vi "Day 5.vi"() -> ()   [LabVIEW 2019]
panel:
  out "Total Time":dbl
  out "Minimize Polymer Time":dbl
  out "React Polymer Time":dbl
  out "Read File Time":dbl
  out "Redux Polymer":string
  out "Error Out":errorcluster
  out "Length of Shortest Polymer":i32
  out "Element Creating Shortest Polymer":string
  out "Polymer Length":i32
  out "Polymer After Reacting":string
  in  "error in (no error)":errorcluster
  in  "Use Example Input":bool
  in  "Example Input":string="dabAcCaCBAcCcaDA"
  in  "Relative Path to Input File":string="Day 5\\Day 5 Raw Input.txt"
  # "Part 1"
  # "Part 2"
  # "~0.43 s is fastest time"
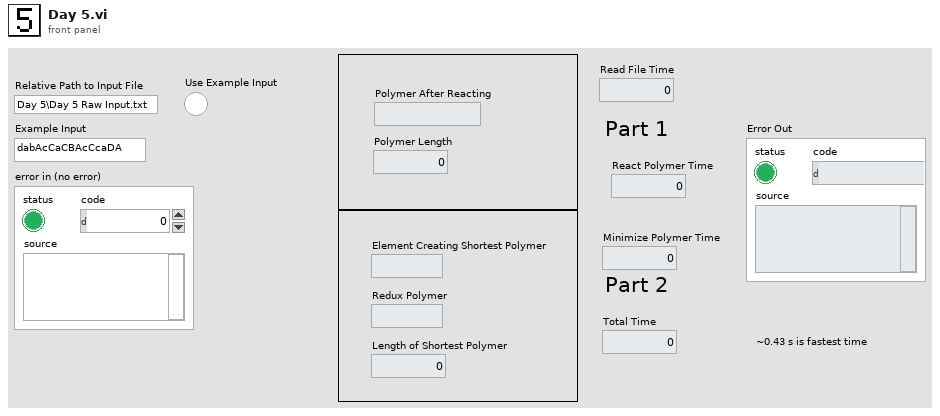
[diagram p1: front panel]
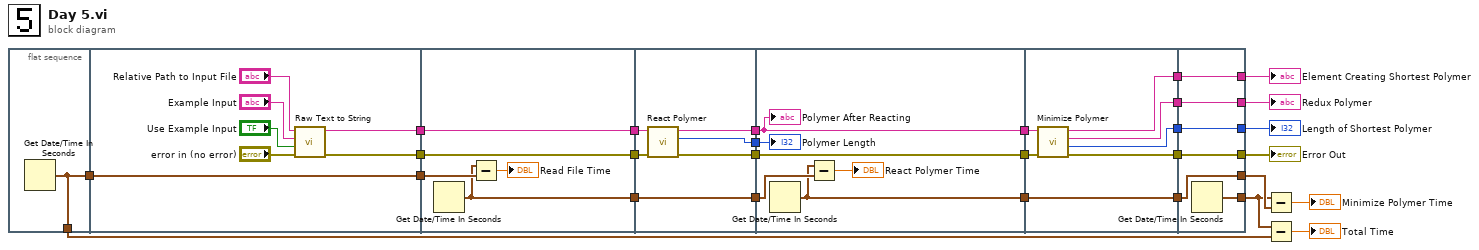
[diagram p0: block diagram]
diagram:
  n1 = flat-sequence {
    tunnel: [w29] -> w28
    tunnel: [w29] -> w9
    tunnel: w28 -> [w36]
    tunnel: [w36] -> w27
    tunnel: [w31] -> w20
    tunnel: [w30] -> w17
    tunnel: w27 -> [w40]
    tunnel: [w39] -> w26
    tunnel: [w38] -> w21
    tunnel: w20 -> [w38]
    tunnel: w17 -> [w37]
    tunnel: [w37] -> w16
    tunnel: w26 -> [w47]
    tunnel: [w47] -> w25
    tunnel: w21 -> [w46]
    tunnel: [w45] -> w19
    tunnel: w16 -> [w44]
    tunnel: [w43] -> w11
    tunnel: [w42] -> w10
    tunnel: w25 -> [w53]
    tunnel: [w51] -> w24
    tunnel: w19 -> [w50]
    tunnel: [w50] -> w18
    tunnel: w11 -> [w49]
    tunnel: w10 -> [w48]
    tunnel: [w48] -> w1
    tunnel: w24 -> [w60]
    tunnel: w18 -> [w59]
    tunnel: [w60] -> w8
    tunnel: [w58] -> w7
    tunnel: [w57] -> w6
    tunnel: [w56] -> w5
    tunnel: [w55] -> w4
    tunnel: w1 -> [w54]
    tunnel: [w62] -> w12
    tunnel: [w63] -> w13
    tunnel: [w64] -> w14
    tunnel: [w65] -> w15
    tunnel: [w66] -> w22
    tunnel: w8 -> [w66]
    tunnel: w7 -> [w65]
    tunnel: w6 -> [w64]
    tunnel: w5 -> [w63]
    tunnel: w4 -> [w62]
    tunnel: [w61] -> w3
    frame #0 {
      n2 = Get Date/Time In Seconds() -> (seconds since 1Jan1904=w29:timestamp)
    }
    frame #1 {
      n3 = call "Raw Text to String.vi"("Error In"="error in (no error)", "Use Example Input"="Use Example Input", "Example Input"="Example Input", "Relative Path to Input File"="Relative Path to Input File") -> ("Error Out"=w30:errorcluster, "String"=w31:string)  [unwired: 6 in]
    }
    frame #2 {
      n4 = Get Date/Time In Seconds() -> (seconds since 1Jan1904=w39:timestamp)
      n5 = Subtract(x=w39, y=w40) -> (x-y=→"Read File Time":dbl)
    }
    frame #3 {
      n6 = call "React Polymer.vi"("Error In"=w44, "Unreacted Polymer"=w46) -> ("Error Out"=w45:errorcluster, "Size of Polymer"=w43:i32, "Polymer"=w42:string)  [unwired: 7 in]
    }
    frame #4 {
      n7 = Get Date/Time In Seconds() -> (seconds since 1Jan1904=w51:timestamp)
      n8 = Subtract(x=w51, y=w53) -> (x-y=→"React Polymer Time":dbl)
      "Polymer Length" <- w49
      "Polymer After Reacting" <- w48
    }
    frame #5 {
      n9 = call "Minimize Polymer.vi"("Error In"=w59, "Unreacted Polymer"=w54) -> ("Error Out"=w55:errorcluster, "Size of Redux Polymer"=w56:i32, "Redux Polymer"=w57:string, "Redux Element"=w58:string)  [unwired: 6 in]
    }
    frame #6 {
      n10 = Get Date/Time In Seconds() -> (seconds since 1Jan1904=w61:timestamp)
    }
  }
  n11 = Subtract(x=w3, y=w22) -> (x-y=→"Minimize Polymer Time":dbl)
  n12 = Subtract(x=w3, y=w9) -> (x-y=→"Total Time":dbl)
  "Element Creating Shortest Polymer" <- w15
  "Length of Shortest Polymer" <- w13
  "Error Out" <- w12
  "Redux Polymer" <- w14
